vi "Application Path.vi"(11 "name or relative path":path) -> (3 "appended path":path)   [LabVIEW 2021]
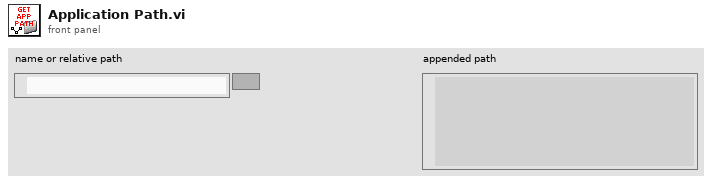
[diagram p1: front panel]
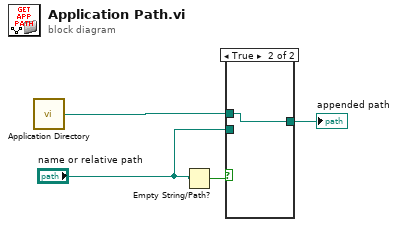
[diagram p0: block diagram]
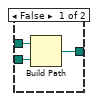
[diagram p2: hidden frame]
diagram:
  n1 = call <vilib>:"Application Directory.vi"() -> ("Application Directory"=w4:path)
  n2 = Empty String/Path?(string/path="name or relative path") -> (empty?=w1:bool)
  n3 = case shown="True" w1 {
    tunnel: w4 -> [w7 w8]
    tunnel: [w6 w8] -> w3
    tunnel: "name or relative path" -> [w5 _]
    frame False {
      n4 = Build Path(base path=w7, name or relative path=w5) -> (appended path=w6:path)
    }
    frame True {
    }
  }
  "appended path" <- w3
